vi "Close.vi"(8 "error in (no error)":errorcluster, 11 "LINX-AutomationHat in":refnum<class "LINX-AutomationHat.lvclass">) -> (0 "error out":errorcluster, 3 "LINX-AutomationHat out":refnum<class "LINX-AutomationHat.lvclass">)   [LabVIEW 2020, in "LINX-AutomationHat.lvclass"]
uses:
  LINX-AutomationHat.lvclass
  LINX-SN3218/LINX-SN3218.lvclass
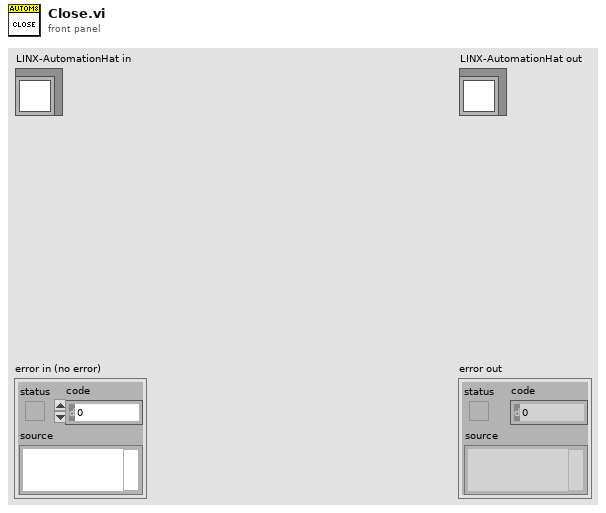
[diagram p1: front panel]
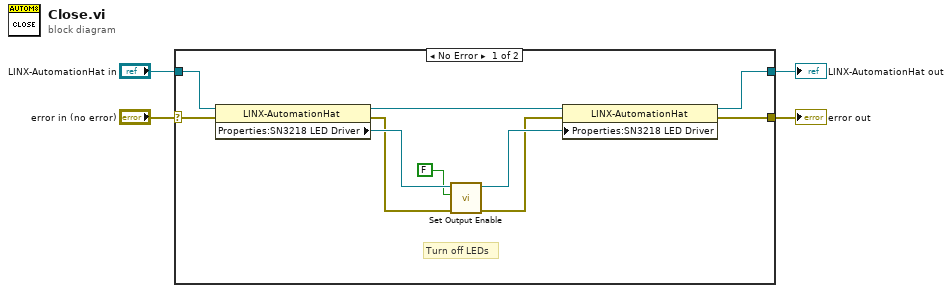
[diagram p0: block diagram]
diagram:
  n1 = case shown="No Error" "error in (no error)" {
    selector: "error in (no error)" -> [w8 w16]
    tunnel: [w5 w16] -> w3
    tunnel: [w10 w15] -> w1
    tunnel: "LINX-AutomationHat in" -> [w14 w15]
    frame No Error {
      # "Turn off LEDs"
      n2 = property class="LINX-AutomationHat"(reference=w14, error in=w8) -> (reference out=w11:refnum<class "LINX-AutomationHat.lvclass">, error out=w7:errorcluster, "Properties:SN3218 LED Driver"=w13:refnum<class "LINX-SN3218.lvclass">)
      n3 = call "Set Output Enable.vi"("error in (no error)"=w7, "Enabled?"=FALSE, "LINX-SN3218 in"=w13) -> ("error out"=w6:errorcluster, "LINX-SN3218 out"=w9:refnum<class "LINX-SN3218.lvclass">)  [unwired: 7 in]
      n4 = property class="LINX-AutomationHat"(reference=w11, error in=w6, "Properties:SN3218 LED Driver"=w9) -> (reference out=w10:refnum<class "LINX-AutomationHat.lvclass">, error out=w5:errorcluster)
    }
    frame Error {
    }
  }
  "error out" <- w3
  "LINX-AutomationHat out" <- w1
